vi "Simple Resample.vi"(9 "sample rate (S/s)":dbl=1.0, 10 "coerced IQ Rate":dbl=1.0, 11 "input waveform":waveform(dbl)) -> (3 "output waveform":waveform(dbl))   [LabVIEW 2015]
uses:
  <vilib>/Analysis/2dsp.llb/Rational Resample (single channel, DBL).vi
  <vilib>/Analysis/NI_AALPro.lvlib
panel:
  out "size(s) 2":i32
  out "size(s)":i32
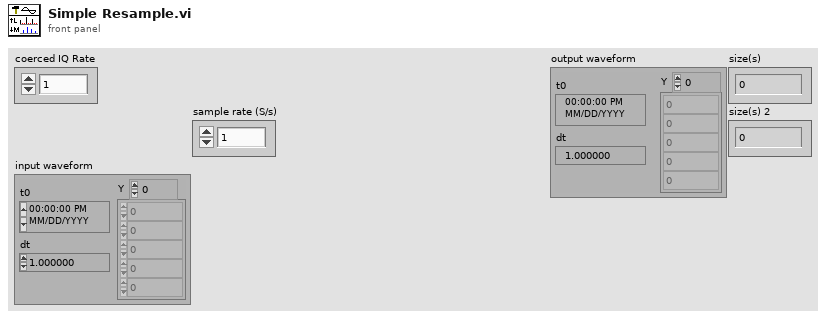
[diagram p1: front panel]
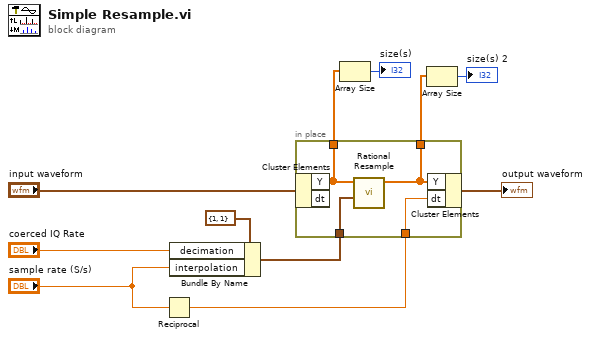
[diagram p0: block diagram]
diagram:
  n1 = Reciprocal(x="sample rate (S/s)") -> (1/x=w6:dbl)
  n2 = Bundle By Name(cluster=cluster{"interpolation":i32, "decimation":i32} {"interpolation"=1, "decimation"=1} ("resample factor"), "decimation"="coerced IQ Rate", "interpolation"="sample rate (S/s)") -> (w7:cluster{"interpolation":i32, "decimation":i32})
  n3 = in-place "In Place Element Structure" {
    in-place-border: w7 -> [w15]
    in-place-border: w6 -> [w14]
    in-place-border: [w13] -> w5
    in-place-border: [w12] -> w4
    n4 = in-place-cluster #1("input waveform") -> ("Y"=w12:dbl[])  [unwired: 1 out]
    n5 = call-poly <vilib>:"Rational Resample.vi"("resample factor"=w15, "X"=w12) -> ("Y"=w13:dbl[])  [unwired: 7 in, 2 out]
    n6 = in-place-cluster #1("Y"=w13, "dt"=w14) -> (→"output waveform":waveform(dbl))
  }
  n7 = Array Size(array=w4) -> (size(s)=→"size(s)":i32)
  n8 = Array Size(array=w5) -> (size(s)=→"size(s) 2":i32)
